vi "Get Category.vi"(8 "error in (no error)":errorcluster, 11 "J1939 editor node in":refnum<class "J1939 editor node.lvclass">) -> (0 "error out":errorcluster, 2 "Category":string, 3 "J1939 editor node out":refnum<class "J1939 editor node.lvclass">)   [LabVIEW 2017, in "J1939 editor node.lvclass"]
uses:
  J1939 editor node.lvclass
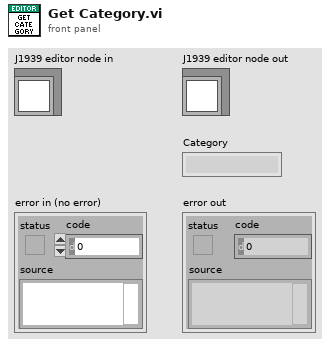
[diagram p1: front panel]
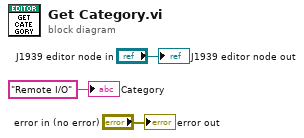
[diagram p0: block diagram]
diagram:
  "error out" <- "error in (no error)"
  "J1939 editor node out" <- "J1939 editor node in"
  "Category" <- "Remote I/O" ("Category")
